vi "Report Main.vi"() -> ()   [LabVIEW 2014]
uses:
  <vilib>/addons/_office/_wordsub.llb/font.ctl
  States1.ctl
panel:
  in  "生成":bool
  in  "取消":bool
  in  "前一项":bool
  in  "后一项":bool
  in  "输出簇":T2={"标题配置"={"title"="测试报告", "font"={"font name"="", "font size"=24.0, "bold"=2, "italic"=2, "underline"=2, "strike through"=2, "font color"=16777222}}, "测试信息"={"font"={"font name"="", "font size"=12.0, "bold"=2, "italic"=2, "underline"=2, "strike through"=2, "font color"=16777222}, "字符串"="时间：8:40 AM\n日期： 9/19/2007\n测试人： 测试人1"}, "文本"={"font"={"font name"="", "font size"=12.0, "bold"=2, "italic"=2, "underline"=2, "strike through"=2, "font color"=16777222}, "字符串"="报告概述：\n        这是一个测试报表，可以生三种不同类型的报表，包括：Html、Word、Excel三种。点击报告类型进行选择。\n        报表分成5个部分：标题，信息，文本，表哥和图表，在\n相应区域双击能够配置前四个部分，在表格区域单击还可以配置图表。\n       点击生成按钮后，报表可以打开并显示。勾选复选框，还可以进行保存、打印、发送E-mail的操作。"}, "表格"={"auto format"=11, "font"={"font name"="", "font size"=12.0, "bold"=2, "italic"=2, "underline"=2, "strike through"=2, "font color"=0}, "表格 2"=[["1", "1.5", "5.6", "5.6", "7.9", "4.6"], ["2", "2.5", "7.6", "6.5", "7.2", "7.5"], ["3", "6.8", "9.1", "4.2", "6.2", "6.1"], ["4", "6.7", "7.1", "7.2", "1.0", "8.3"], ["5", "6.4", "4.3", "9.2", "5.8", "4.2"], ["6", "8.6", "8.2", "4.3", "8.6", "4.5"]]}, "图表配置"={"chart type"=4, "graph title (\"\")"="测试图表"}, "保存设置"={"Save Report 2"=FALSE, "路径"=path "H:/Report.html", "Print Report 2"=FALSE, "份数"=1}, "报告类型"=0} {"保存设置"."份数" min=1 max=10 step=1; "图表配置"."chart type" items=["xlColumnClustered"=51, "xlColumnStacked"=52, "xlColumnStacked100"=53, "xl3DColumnClustered"=54, "xl3DColumnStacked"=55, "xl3DColumnStacked100"=56, "xlBarClustered"=57, "xlBarStacked"=58, "xlBarStacked100"=59, "xl3DBarClustered"=60, "xl3DBarStacked"=61, "xl3DBarStacked100"=62, "xlLineStacked"=63, "xlLineStacked100"=64, "xlLineMarkers"=65, "xlLineMarkersStacked"=66, "xlLineMarkersStacked100"=67, "xlPieOfPie"=68, "xlPieExploded"=69, "xl3DPieExploded"=70, "xlBarOfPie"=71, "xlXYScatterSmooth"=72, "xlXYScatterSmoothNoMarkers"=73, "xlXYScatterLines"=74, "xlXYScatterLinesNoMarkers"=75, "xlAreaStacked"=76, "xlAreaStacked100"=77, "xl3DAreaStacked"=78, "xl3DAreaStacked100"=79, "xlDoughnutExploded"=80, "xlRadarMarkers"=81, "xlRadarFilled"=82, "xlSurface"=83, "xlSurfaceWireframe"=84, "xlSurfaceTopView"=85, "xlSurfaceTopViewWireframe"=86, "xlBubble"=15, "xlBubble3DEffect"=87, "xlStockHLC"=88, "xlStockOHLC"=89, "xlStockVHLC"=90, "xlStockVOHLC"=91, "xlCylinderColClustered"=92, "xlCylinderColStacked"=93, "xlCylinderColStacked100"=94, "xlCylinderBarClustered"=95, "xlCylinderBarStacked"=96, "xlCylinderBarStacked100"=97, "xlCylinderCol"=98, "xlConeColClustered"=99, "xlConeColStacked"=100, "xlConeColStacked100"=101, "xlConeBarClustered"=102, "xlConeBarStacked"=103, "xlConeBarStacked100"=104, "xlConeCol"=105, "xlPyramidColClustered"=106, "xlPyramidColStacked"=107, "xlPyramidColStacked100"=108, "xlPyramidBarClustered"=109, "xlPyramidBarStacked"=110, "xlPyramidBarStacked100"=111, "xlPyramidCol"=112, "xl3DColumn"=-4100, "xlLine"=4, "xl3DLine"=-4101, "xl3DPie"=-4102, "xlPie"=5, "xlXYScatter"=-4169, "xl3DArea"=-4098, "xlArea"=1, "xlDoughnut"=-4120, "xlRadar"=-4151]; "表格"."font"."font size" format="%0.2f"; "表格"."font"."strike through" items=["Unchanged", "Yes", "No"]; "表格"."font"."underline" items=["Unchanged", "Yes", "No"]; "表格"."font"."italic" items=["Unchanged", "Yes", "No"]; "表格"."font"."bold" items=["Unchanged", "Yes", "No"]; "表格"."auto format" items=["xlRangeAutoFormat3DEffects1"=13, "xlRangeAutoFormat3DEffects2"=14, "xlRangeAutoFormatAccounting1"=4, "xlRangeAutoFormatAccounting2"=5, "xlRangeAutoFormatAccounting3"=6, "xlRangeAutoFormatAccounting4"=17, "xlRangeAutoFormatClassic1"=1, "xlRangeAutoFormatClassic2"=2, "xlRangeAutoFormatClassic3"=3, "xlRangeAutoFormatColor1"=7, "xlRangeAutoFormatColor2"=8, "xlRangeAutoFormatColor3"=9, "xlRangeAutoFormatList1"=10, "xlRangeAutoFormatList2"=11, "xlRangeAutoFormatList3"=12, "xlRangeAutoFormatLocalFormat1"=15, "xlRangeAutoFormatLocalFormat2"=16, "xlRangeAutoFormatLocalFormat3"=19, "xlRangeAutoFormatLocalFormat4"=20, "xlRangeAutoFormatReport1"=21, "xlRangeAutoFormatReport2"=22, "xlRangeAutoFormatReport3"=23, "xlRangeAutoFormatReport4"=24, "xlRangeAutoFormatReport5"=25, "xlRangeAutoFormatReport6"=26, "xlRangeAutoFormatReport7"=27, "xlRangeAutoFormatReport8"=28, "xlRangeAutoFormatReport9"=29, "xlRangeAutoFormatReport10"=30, "xlRangeAutoFormatClassicPivotTable"=31, "xlRangeAutoFormatTable1"=32, "xlRangeAutoFormatTable2"=33, "xlRangeAutoFormatTable3"=34, "xlRangeAutoFormatTable4"=35, "xlRangeAutoFormatTable5"=36, "xlRangeAutoFormatTable6"=37, "xlRangeAutoFormatTable7"=38, "xlRangeAutoFormatTable8"=39, "xlRangeAutoFormatTable9"=40, "xlRangeAutoFormatTable10"=41, "xlRangeAutoFormatPTNone"=42, "xlRangeAutoFormatNone"=-4142, "xlRangeAutoFormatSimple"=-4154]; "文本"."font"."font size" format="%0.2f"; "文本"."font"."strike through" items=["Strk Unchanged", "Strk Yes", "Strk No"]; "文本"."font"."underline" items=["Und Unchanged", "Und Yes", "Und No"]; "文本"."font"."italic" items=["Ital Unchanged", "Ital Yes", "Ital No"]; "文本"."font"."bold" items=["Bold Unchanged", "Bold Yes", "Bold No"]; "测试信息"."font"."font size" format="%0.2f"; "测试信息"."font"."strike through" items=["Strk Unchanged", "Strk Yes", "Strk No"]; "测试信息"."font"."underline" items=["Und Unchanged", "Und Yes", "Und No"]; "测试信息"."font"."italic" items=["Ital Unchanged", "Ital Yes", "Ital No"]; "测试信息"."font"."bold" items=["Bold Unchanged", "Bold Yes", "Bold No"]; "标题配置"."font"."font size" format="%0.2f"; "标题配置"."font"."strike through" items=["Unchanged", "Yes", "No"]; "标题配置"."font"."underline" items=["Unchanged", "Yes", "No"]; "标题配置"."font"."italic" items=["Unchanged", "Yes", "No"]; "标题配置"."font"."bold" items=["Unchanged", "Yes", "No"]}
  out "选项卡控件":enum32{"报告界面", "报告属性", "报告参数"}(tab)
  in  "介绍":string="报告概述：\n        这是一个测试报表，可以生三种不同类型的报表，包括：Html、Word、Excel三种。\n        报表分成5个部分：标题，信息，文本，表格以及图表。 \n        点击生成按钮后，报表可以打开并显示。\n        请点击向右的箭头进行下一步操作。"
  in  "表格":string[][](table)=[["1", "1.5", "5.6", "5.6", "7.9", "4.6"], ["2", "2.5", "7.6", "6.5", "7.2", "7.5"], ["3", "6.8", "9.1", "4.2", "6.2", "6.1"], ["4", "6.7", "7.1", "7.2", "1.0", "8.3"], ["5", "6.4", "4.3", "9.2", "5.8", "4.2"], ["6", "8.6", "8.2", "4.3", "8.6", "4.5"]]
  in  "测试者":string="测试人1"
  out "时间":string="8:40 AM"
  out "日期":string="9/19/2007"
  in  "标题":string="测试报告"
  in  "保存":bool
  in  "打印":bool
  in  "路径":path=path "H:/Report.html"
  in  "份数":i32=1 min=1 max=10 step=1
  in  "报告类型":u16(ring)
  in  "字号 2":dbl=24.0
  in  "粗体":u16(ring)=2 items=["Yes"=1, "No"=2]
  in  "字号":dbl=12.0
  in  "下划线":u16(ring)=2 items=["Yes"=1, "No"=2]
  in  "字号":dbl=12.0
  in  "字号":dbl=12.0
  in  "表格格式":i32(ring)=11 items=["格式1", "格式2", "格式3", "格式4", "格式5", "格式6", "格式7", "格式8", "格式9", "格式10", "格式11", "格式12", "格式13", "格式14", "格式15", "格式16"]
  in  "图表标题":string="测试图表"
  in  "图表类型":i32(ring)=4 items=["xlColumnClustered"=51, "xlColumnStacked"=52, "xlColumnStacked100"=53, "xl3DColumnClustered"=54, "xl3DColumnStacked"=55, "xl3DColumnStacked100"=56, "xlBarClustered"=57, "xlBarStacked"=58, "xlBarStacked100"=59, "xl3DBarClustered"=60, "xl3DBarStacked"=61, "xl3DBarStacked100"=62, "xlLineStacked"=63, "xlLineStacked100"=64, "xlLineMarkers"=65, "xlLineMarkersStacked"=66, "xlLineMarkersStacked100"=67, "xlPieOfPie"=68, "xlPieExploded"=69, "xl3DPieExploded"=70, "xlBarOfPie"=71, "xlXYScatterSmooth"=72, "xlXYScatterSmoothNoMarkers"=73, "xlXYScatterLines"=74, "xlXYScatterLinesNoMarkers"=75, "xlAreaStacked"=76, "xlAreaStacked100"=77, "xl3DAreaStacked"=78, "xl3DAreaStacked100"=79, "xlDoughnutExploded"=80, "xlRadarMarkers"=81, "xlRadarFilled"=82, "xlSurface"=83, "xlSurfaceWireframe"=84, "xlSurfaceTopView"=85, "xlSurfaceTopViewWireframe"=86, "xlBubble"=15, "xlBubble3DEffect"=87, "xlStockHLC"=88, "xlStockOHLC"=89, "xlStockVHLC"=90, "xlStockVOHLC"=91, "xlCylinderColClustered"=92, "xlCylinderColStacked"=93, "xlCylinderColStacked100"=94, "xlCylinderBarClustered"=95, "xlCylinderBarStacked"=96, "xlCylinderBarStacked100"=97, "xlCylinderCol"=98, "xlConeColClustered"=99, "xlConeColStacked"=100, "xlConeColStacked100"=101, "xlConeBarClustered"=102, "xlConeBarStacked"=103, "xlConeBarStacked100"=104, "xlConeCol"=105, "xlPyramidColClustered"=106, "xlPyramidColStacked"=107, "xlPyramidColStacked100"=108, "xlPyramidBarClustered"=109, "xlPyramidBarStacked"=110, "xlPyramidBarStacked100"=111, "xlPyramidCol"=112, "xl3DColumn"=-4100, "xlLine"=4, "xl3DLine"=-4101, "xl3DPie"=-4102, "xlPie"=5, "xlXYScatter"=-4169, "xl3DArea"=-4098, "xlArea"=1, "xlDoughnut"=-4120, "xlRadar"=-4151]
  # "报告界面"
  # "配置区域"
  # "标   题"
  # "测试信息"
  # "文   本"
  # "表   格"
  # "图   表"
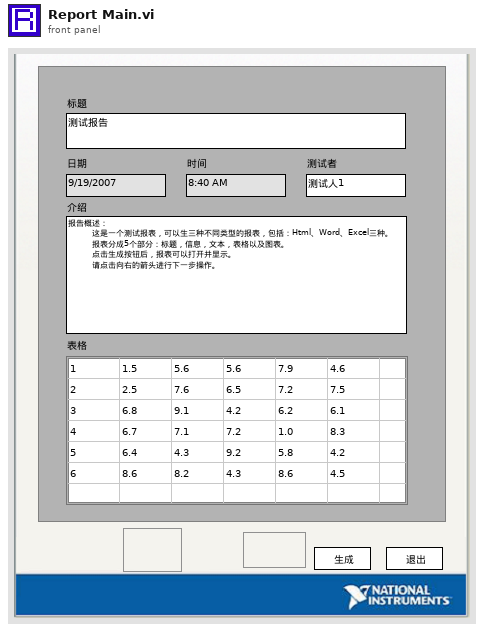
[diagram p1: front panel]
types:
  T1 = typedef "font.ctl" = cluster{"font name":string, "font size":dbl, "bold":u16, "italic":u16, "underline":u16, "strike through":u16, "font color":u32}
  T2 = cluster{"标题配置":cluster{"title":string, "font":T1}, "测试信息":cluster{"font":T1, "字符串":string}, "文本":cluster{"font":T1, "字符串":string}, "表格":cluster{"auto format":i32, "font":T1, "表格 2":string[][]}, "图表配置":cluster{"chart type":i32, "graph title (\"\")":string}, "保存设置":cluster{"Save Report 2":bool, "路径":path, "Print Report 2":bool, "份数":i32}, "报告类型":u16}
  T3 = typedef "States1.ctl" = enum16{"初始化", "等待", "捆绑参数", "生成", "停止"}
  T4 = cluster{"auto format":i32, "font":T1, "表格 2":string[][]}
  T5 = cluster{"chart type":i32, "graph title (\"\")":string}
  T6 = cluster{"Save Report 2":bool, "路径":path, "Print Report 2":bool, "份数":i32}
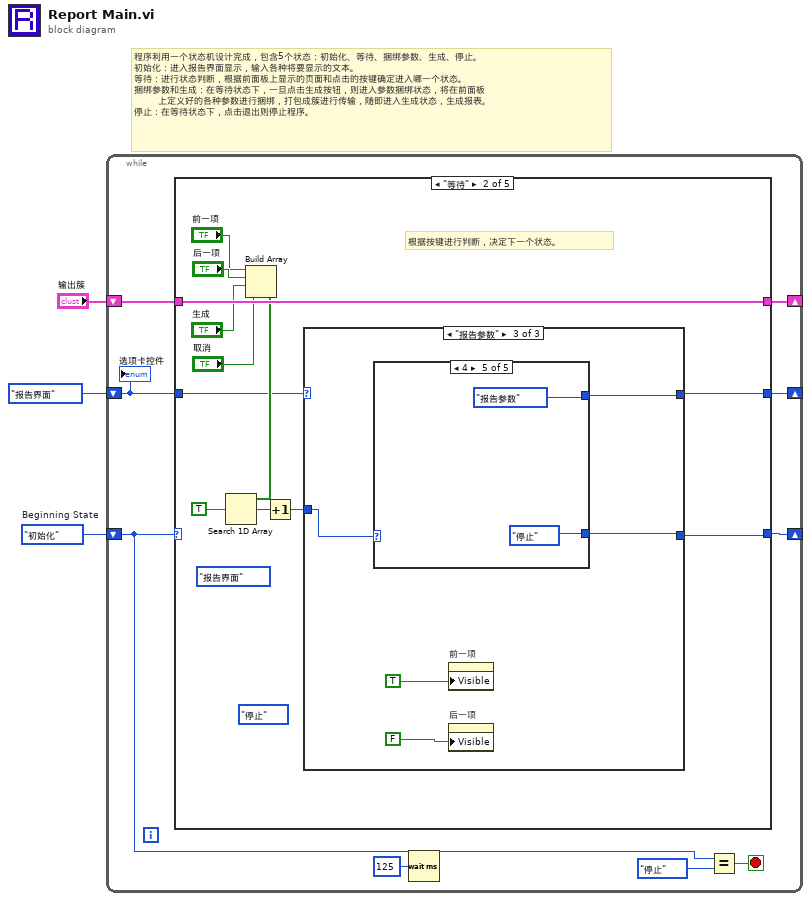
[diagram p0: block diagram]
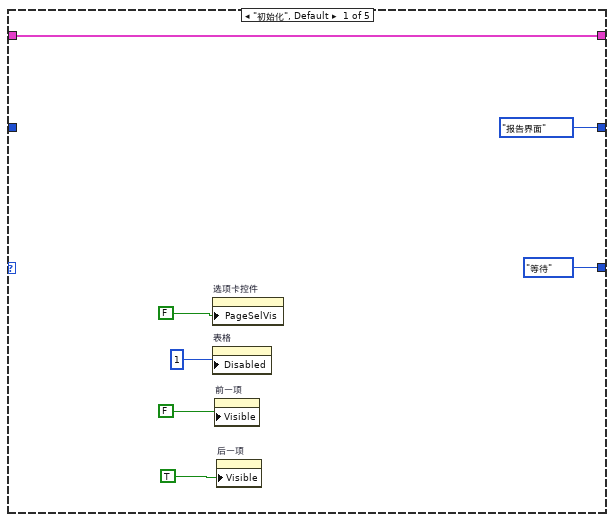
[diagram p2: hidden frame]
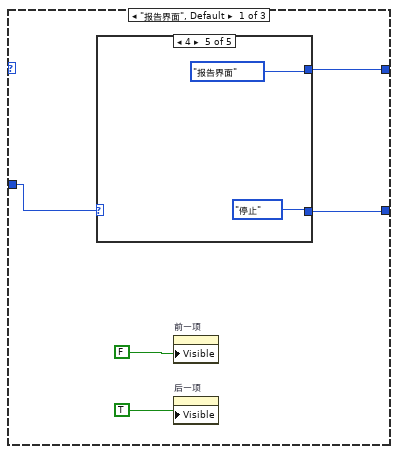
[diagram p3: hidden frame]
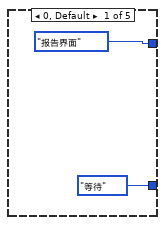
[diagram p4: hidden frame]
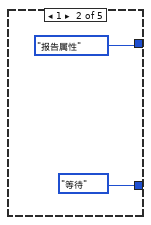
[diagram p5: hidden frame]
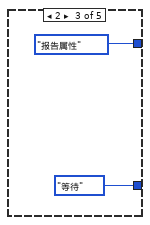
[diagram p6: hidden frame]
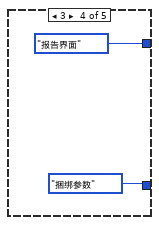
[diagram p7: hidden frame]
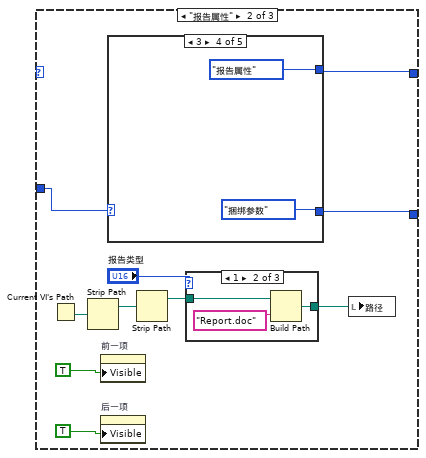
[diagram p8: hidden frame]
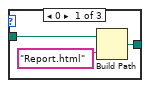
[diagram p9: hidden frame]
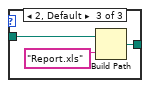
[diagram p10: hidden frame]
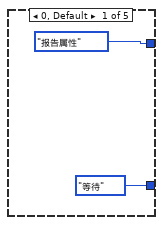
[diagram p11: hidden frame]
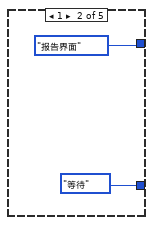
[diagram p12: hidden frame]
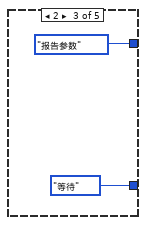
[diagram p13: hidden frame]
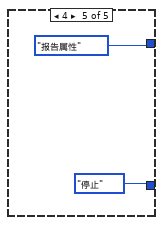
[diagram p14: hidden frame]
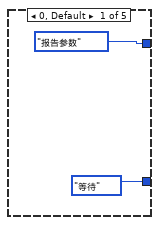
[diagram p15: hidden frame]
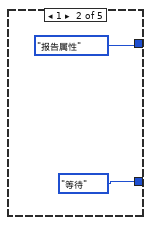
[diagram p16: hidden frame]
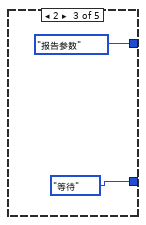
[diagram p17: hidden frame]
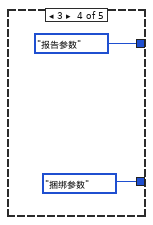
[diagram p18: hidden frame]
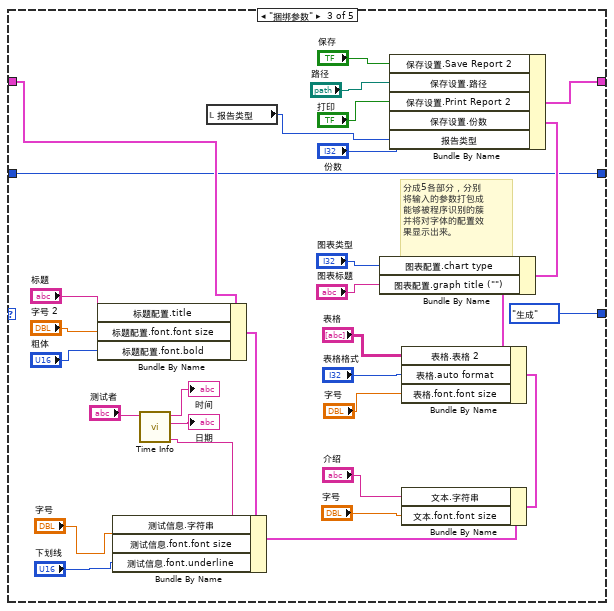
[diagram p19: hidden frame]
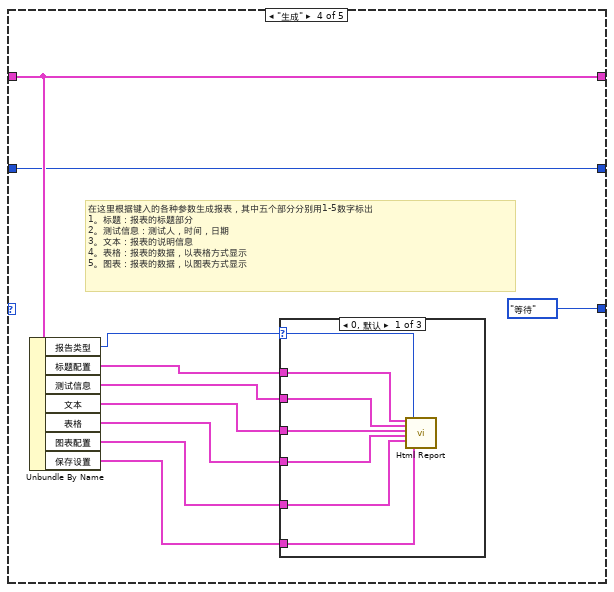
[diagram p20: hidden frame]
diagram:
  w3 = States1."初始化"  # Beginning State
  # "程序利用一个状态机设计完成，包含5个状态：初始化、等待、捆绑参数、生成、停止。\n初始化：进入报告界面显示，输入各种将要显示的文本。\n等待：进行状态判断，根据前面板上显示的页面和点击的按键确定进入哪一个状态。\n捆绑参数和生成：在等待状态下，一旦点击生成按钮，则进入参数捆绑状态，将在前面板\n        上定义好的各种参数进行捆绑，打包成簇进行传输，随即进入生成状态，生成报表。\n停止：在等待状态下，点击退出则停止程序。"
  n1 = while {
    shift-right: [w10] -> _
    shift-left: w3 -> [w11]
    shift-right: [w7] -> _
    shift-left: "输出簇" -> [w6]
    shift-right: [w4] -> _
    shift-left: enum32{"报告界面", "报告属性", "报告参数"}."报告界面" ("选项卡控件") -> [w5]
    stop <- w12 stop-if-true
    n2 = case shown="\"等待\"" w11 {
      tunnel: [States1."等待" ("States") w22 States1."生成" ("States") States1."等待" ("States") States1."停止" ("States")] -> w10
      tunnel: [w17 w31 w96 w129 w153] -> w7
      tunnel: w6 -> [w17 w31 w120 w129 w153]
      tunnel: w5 -> [_ w23 w94 w121 w152]
      tunnel: [enum32{"报告界面", "报告属性", "报告参数"}."报告界面" ("选项卡控件") w24 w94 w121 w152] -> w4
      frame "初始化", Default {
        n3 = property on="选项卡控件" class="TabCtl (严格)"("PageSelVis"=FALSE ("页选择器可见")) -> ()  [unwired: 2 in, 2 out]
        n4 = property on="表格" class="Tbl (严格)"("Disabled"=u8 1 ("禁用")) -> ()  [unwired: 2 in, 2 out]
        n5 = property on="前一项" class="Bool"("Visible"=FALSE ("可见")) -> ()  [unwired: 2 in, 2 out]
        n6 = property on="后一项" class="Bool"("Visible"=TRUE ("可见")) -> ()  [unwired: 2 in, 2 out]
      }
      frame "等待" {
        (unwired) States1."停止" ("States")
        (unwired) enum32{"报告界面", "报告属性", "报告参数"}."报告界面" ("选项卡控件")
        # "根据按键进行判断，决定下一个状态。"
        n7 = Build Array("前一项", "后一项", "生成", "取消") -> (w26:bool[])
        n8 = Search 1D Array(1D array=w26, element=TRUE ("元素")) -> (index of element=w21:i32)  [unwired: 1 in]
        n9 = Increment(x=w21) -> (x+1=w20:i32)
        n10 = case shown="\"报告参数\"" w23 {
          tunnel: [w33 w52 w77] -> w22
          tunnel: [w32 w53 w78] -> w24
          tunnel: w20 -> [w34 w54 w76]
          frame "报告界面", Default {
            n11 = case shown="4" w34 {
              tunnel: [States1."等待" ("States") States1."等待" ("States") States1."等待" ("States") States1."捆绑参数" ("States") States1."停止" ("States")] -> w33
              tunnel: [enum32{"报告界面", "报告属性", "报告参数"}."报告界面" ("选项卡控件") enum32{"报告界面", "报告属性", "报告参数"}."报告属性" ("选项卡控件") enum32{"报告界面", "报告属性", "报告参数"}."报告属性" ("选项卡控件") enum32{"报告界面", "报告属性", "报告参数"}."报告界面" ("选项卡控件") enum32{"报告界面", "报告属性", "报告参数"}."报告界面" ("选项卡控件")] -> w32
              frame 0, Default {
              }
              frame 1 {
              }
              frame 2 {
              }
              frame 3 {
              }
              frame 4 {
              }
            }
            n12 = property on="前一项" class="Bool"("Visible"=FALSE ("可见")) -> ()  [unwired: 2 in, 2 out]
            n13 = property on="后一项" class="Bool"("Visible"=TRUE ("可见")) -> ()  [unwired: 2 in, 2 out]
          }
          frame "报告属性" {
            n14 = Current VI's Path() -> (path=w50:path)
            n15 = Strip Path(path=w50) -> (stripped path=w51:path)  [unwired: 1 out]
            n16 = property on="前一项" class="Bool"("Visible"=TRUE ("可见")) -> ()  [unwired: 2 in, 2 out]
            n17 = property on="后一项" class="Bool"("Visible"=TRUE ("可见")) -> ()  [unwired: 2 in, 2 out]
            n18 = case shown="3" w54 {
              tunnel: [States1."等待" ("States") States1."等待" ("States") States1."等待" ("States") States1."捆绑参数" ("States") States1."停止" ("States")] -> w52
              tunnel: [enum32{"报告界面", "报告属性", "报告参数"}."报告属性" ("选项卡控件") enum32{"报告界面", "报告属性", "报告参数"}."报告界面" ("选项卡控件") enum32{"报告界面", "报告属性", "报告参数"}."报告参数" ("选项卡控件") enum32{"报告界面", "报告属性", "报告参数"}."报告属性" ("选项卡控件") enum32{"报告界面", "报告属性", "报告参数"}."报告属性" ("选项卡控件")] -> w53
              frame 0, Default {
              }
              frame 1 {
              }
              frame 2 {
              }
              frame 3 {
              }
              frame 4 {
              }
            }
            n19 = Strip Path(path=w51) -> (stripped path=w49:path)  [unwired: 1 out]
            n20 = case shown="1" "报告类型" {
              tunnel: w49 -> [w58 w61 w64]
              tunnel: [w57 w60 w63] -> w47
              frame 0 {
                n21 = Build Path(base path=w58, name or relative path="Report.html" ("名称或相对路径")) -> (appended path=w57:path)
              }
              frame 1 {
                n22 = Build Path(base path=w61, name or relative path="Report.doc" ("名称或相对路径")) -> (appended path=w60:path)
              }
              frame 2, Default {
                n23 = Build Path(base path=w64, name or relative path="Report.xls" ("名称或相对路径")) -> (appended path=w63:path)
              }
            }
            n24 = local write "路径"(w47) -> ()
          }
          frame "报告参数" {
            n25 = case shown="4" w76 {
              tunnel: [States1."等待" ("States") States1."等待" ("States") States1."等待" ("States") States1."捆绑参数" ("States") States1."停止" ("States")] -> w77
              tunnel: [enum32{"报告界面", "报告属性", "报告参数"}."报告参数" ("选项卡控件") enum32{"报告界面", "报告属性", "报告参数"}."报告属性" ("选项卡控件") enum32{"报告界面", "报告属性", "报告参数"}."报告参数" ("选项卡控件") enum32{"报告界面", "报告属性", "报告参数"}."报告参数" ("选项卡控件") enum32{"报告界面", "报告属性", "报告参数"}."报告参数" ("选项卡控件")] -> w78
              frame 0, Default {
              }
              frame 1 {
              }
              frame 2 {
              }
              frame 3 {
              }
              frame 4 {
              }
            }
            n26 = property on="前一项" class="Bool"("Visible"=TRUE ("可见")) -> ()  [unwired: 2 in, 2 out]
            n27 = property on="后一项" class="Bool"("Visible"=FALSE ("可见")) -> ()  [unwired: 2 in, 2 out]
          }
        }
      }
      frame "捆绑参数" {
        # "分成5各部分，分别\n将输入的参数打包成\n能够被程序识别的簇\n并将对字体的配置效\n果显示出来。"
        n28 = Bundle By Name(cluster=w120, "标题配置.title"="标题", "标题配置.font.font size"="字号 2", "标题配置.font.bold"="粗体") -> (w105:T2)
        n29 = call "Time Info.vi"("测试人"="测试者") -> ("字符串"=w113:string, "日期"=→"日期":string, "时间"=→"时间":string)  [unwired: 7 in, 1 out]
        n30 = Bundle By Name(cluster=w105, "测试信息.字符串"=w113, "测试信息.font.font size"="字号", "测试信息.font.underline"="下划线") -> (w103:T2)
        n31 = local read "报告类型"() -> (w91:u16)
        n32 = Bundle By Name(cluster=w103, "文本.字符串"="介绍", "文本.font.font size"="字号") -> (w101:T2)
        n33 = Bundle By Name(cluster=w101, "表格.表格 2"="表格", "表格.auto format"="表格格式", "表格.font.font size"="字号") -> (w100:T2)
        n34 = Bundle By Name(cluster=w100, "图表配置.chart type"="图表类型", "图表配置.graph title (\"\")"="图表标题") -> (w95:T2)
        n35 = Bundle By Name(cluster=w95, "保存设置.Save Report 2"="保存", "保存设置.路径"="路径", "保存设置.Print Report 2"="打印", "保存设置.份数"="份数", "报告类型"=w91) -> (w96:T2)
      }
      frame "生成" {
        # "在这里根据键入的各种参数生成报表，其中五个部分分别用1-5数字标出\n1。标题：报表的标题部分\n2。测试信息：测试人，时间，日期\n3。文本：报表的说明信息\n4。表格：报表的数据，以表格方式显示\n5。图表：报表的数据，以图表方式显示"
        n36 = Unbundle By Name(w129) -> ("报告类型"=w122:u16, "标题配置"=w128:cluster{"title":string, "font":T1}, "测试信息"=w127:cluster{"font":T1, "字符串":string}, "文本"=w126:cluster{"font":T1, "字符串":string}, "表格"=w125:T4, "图表配置"=w124:T5, "保存设置"=w123:T6)
        n37 = case shown="0, 默认" w122 {
          selector: w122 -> [w132 w139 w151]
          tunnel: w128 -> [w137 w144 w145]
          tunnel: w127 -> [w136 w143 w146]
          tunnel: w124 -> [w135 w140 w149]
          tunnel: w126 -> [w134 w142 w147]
          tunnel: w125 -> [w133 w141 w148]
          tunnel: w123 -> [w131 w138 w150]
          frame 0, Default {
            n38 = call "Html Report.vi"("标题配置"=w137, "测试信息"=w136, "文本"=w134, "表格"=w133, "图表配置"=w135, "报告类型"=w132, "簇"=w131) -> ()  [unwired: 13 in]
          }
          frame 1 {
            n39 = call "Word Report.vi"("标题配置"=w144, "测试信息"=w143, "文本"=w142, "表格"=w141, "图表配置"=w140, "报告类型"=w139, "簇"=w138) -> ()  [unwired: 13 in]
          }
          frame 2 {
            n40 = call "Excel Report.vi"("标题配置"=w145, "测试信息"=w146, "文本"=w147, "表格"=w148, "图表配置"=w149, "报告类型"=w151, "簇"=w150) -> ()  [unwired: 13 in]
          }
        }
      }
      frame "停止" {
      }
    }
    n41 = Wait (ms)(milliseconds to wait=u32 125) -> ()  [unwired: 1 out]
    n42 = Equal?(x=w11, y=States1."停止" ("States")) -> (x = y?=w12:bool)
    "选项卡控件" <- w5
  }
